vi "Trigger.vi"(8 "error in (no error)":errorcluster, 9 "State, Plant 2":dbl[](array[numeric]), 10 "State, Plant 1":dbl[](array[numeric]), 11 "Plant to trigg":enum16{"Plant 1", "Plant 2"}(ring)) -> (0 "error out":errorcluster, 3 "Kx":dbl)   [LabVIEW 2016]
uses:
  <vilib>/xnet/xnet.llb/XNET Write (Signal Single-point).vi
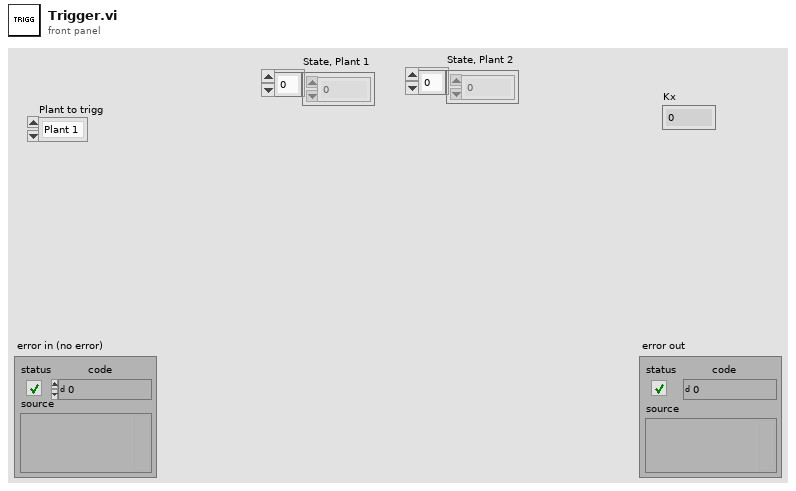
[diagram p1: front panel]
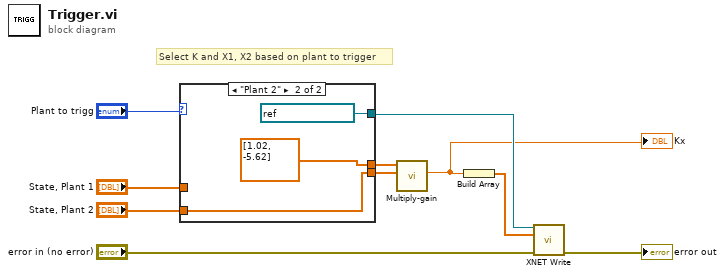
[diagram p0: block diagram]
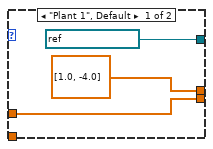
[diagram p2: hidden frame]
diagram:
  # "Select K and X1, X2 based on plant to trigger"
  n1 = case shown="\"Plant 2\"" "Plant to trigg" {
    tunnel: [refnum<k21> "Plant1_Input" ("XNET Session") refnum<k21> "Plant2_Input" ("XNET Session")] -> w8
    tunnel: [dbl[] [1.0, -4.0] ("Gain (K)") dbl[] [1.02, -5.62] ("Gain (K)")] -> w7
    tunnel: [w11 w14] -> w3
    tunnel: "State, Plant 1" -> [w11 _]
    tunnel: "State, Plant 2" -> [_ w14]
    frame "Plant 1", Default {
    }
    frame "Plant 2" {
    }
  }
  n2 = call "Multiply-gain.vi"("State (X)"=w3, "Gain (K)"=w7) -> ("Kx"=w2:dbl)  [unwired: 9 in]
  "Kx" <- w2
  n3 = Build Array(w2) -> (w1:dbl[])
  n4 = call-poly <vilib>:"XNET Write.vi"("session in"=w8, "data"=w1, "error in (no error)"="error in (no error)") -> ("error out"=→"error out":errorcluster)  [unwired: 11 in, 1 out]
